vi "Enclose with Case Structure.vi"(8 "error in (no error)":errorcluster, 11 "VI in":refnum<vi>) -> (0 "error out":errorcluster, 2 "case structure":refnum<vi>, 3 "VI out":refnum<vi>)   [LabVIEW 2017]
uses:
  <vilib>/Utility/traverseref.llb/TRef TravTarget.ctl
  <vilib>/Utility/traverseref.llb/VI Scripting - Traverse.lvlib
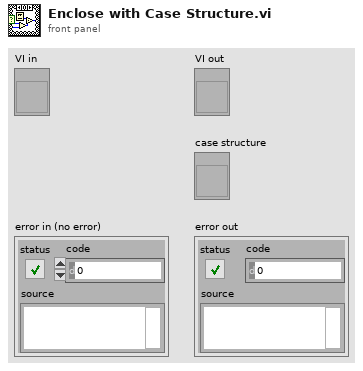
[diagram p1: front panel]
types:
  T1 = typedef "TRef TravTarget.ctl" = enum16{"FP", "BD", "Other"}
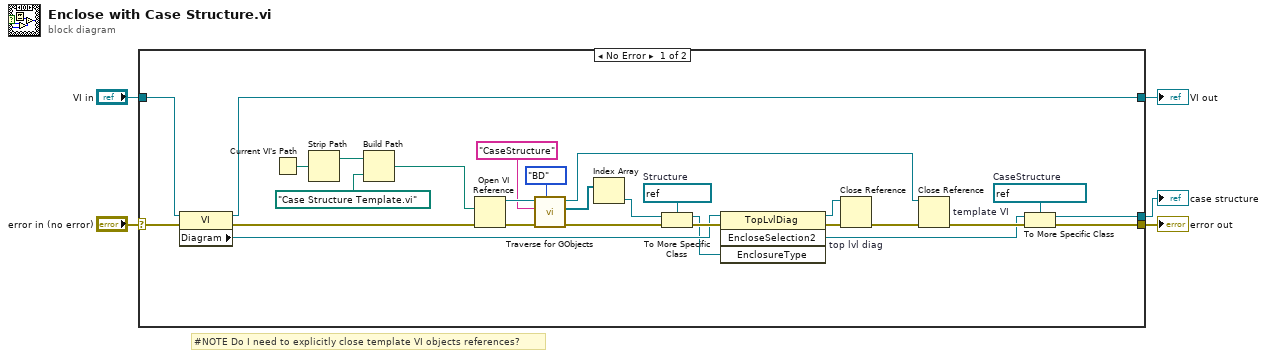
[diagram p0: block diagram]
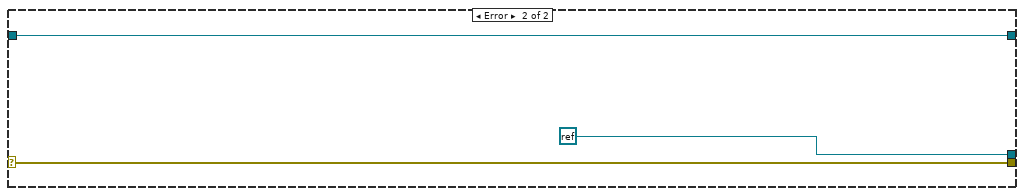
[diagram p2: hidden frame]
diagram:
  # "#NOTE Do I need to explicitly close template VI objects references?"
  n1 = case shown="No Error" "error in (no error)" {
    selector: "error in (no error)" -> [w24 w36]
    tunnel: [w30 w36] -> w5
    tunnel: [w29 refnum<k0> refnum] -> w4
    tunnel: "VI in" -> [w26 w34]
    tunnel: [w14 w34] -> w1
    frame No Error {
      w16 = refnum<vi> refnum  # Structure
      w28 = refnum<vi> refnum  # CaseStructure
      n2 = property class="VI"(reference=w26, error in=w24) -> (reference out=w14:refnum<vi>, error out=w18:errorcluster, "Diagram"=w25:refnum<vi>)
      n3 = Current VI's Path() -> (path=w7:path)
      n4 = Strip Path(path=w7) -> (stripped path=w6:path)  [unwired: 1 out]
      n5 = Build Path(base path=w6, name or relative path=path "Case Structure Template.vi") -> (appended path=w22:path)
      n6 = Open VI Reference(vi path=w22, error in (no error)=w18) -> (vi reference=w21:refnum<vi>, error out=w23:errorcluster)  [unwired: 4 in]
      n7 = call <vilib>:"Traverse for GObjects.vi"("Traverse Target"=TRef_TravTarget."BD", "error in (no error)"=w23, "Class Name"="CaseStructure", "VI Refnum"=w21) -> ("error out"=w15:errorcluster, "References"=w10:refnum<vi>[], "dup VI Refnum"=w9:refnum<vi>)  [unwired: 4 in, 1 out]
      n8 = Index Array(array=w10) -> (element=w17:refnum<vi>)  [unwired: 1 in]
      n9 = To More Specific Class(target class=w16, reference=w17, error in=w15) -> (specific class reference=w11:refnum<vi>, error out=w32:errorcluster)
      n10 = invoke class="TopLvlDiag" method="EncloseSelection2"(reference=w25, error in=w32, "EnclosureType"=w11) -> (reference out=w12:refnum<vi>, error out=w31:errorcluster, "EncloseSelection2"=w27:refnum<vi>)  [unwired: 1 in, 1 out]
      n11 = Close Reference "top lvl diag"(reference=w12, error in (no error)=w31) -> (error out=w13:errorcluster)
      n12 = Close Reference "template VI"(reference=w9, error in (no error)=w13) -> (error out=w33:errorcluster)
      n13 = To More Specific Class(target class=w28, reference=w27, error in=w33) -> (specific class reference=w29:refnum<vi>, error out=w30:errorcluster)
    }
    frame Error {
    }
  }
  "error out" <- w5
  "case structure" <- w4
  "VI out" <- w1
